vi "CC Pressure Monitor Data buffer.vi"(6 "Clear":bool, 8 "error in (no error)":errorcluster, 9 "Write?":bool, 10 "Data":dbl[](array[numeric]), 11 "Time Stamp":timestamp) -> (0 "error out":errorcluster, 3 "XY Graph":T1(graph))   [LabVIEW 2021]
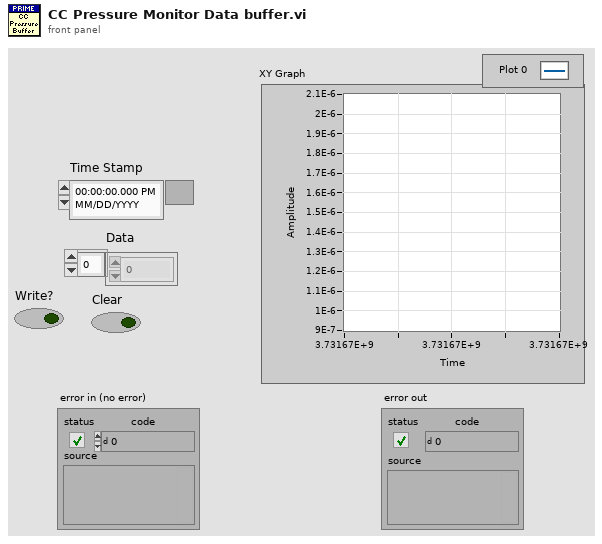
[diagram p1: front panel]
types:
  T1 = cluster{cluster{"Time Stamp":timestamp, "Numeric":dbl}[]}[]
  T2 = cluster{cluster{"Time Stamp":timestamp, "Numeric":dbl}[]}
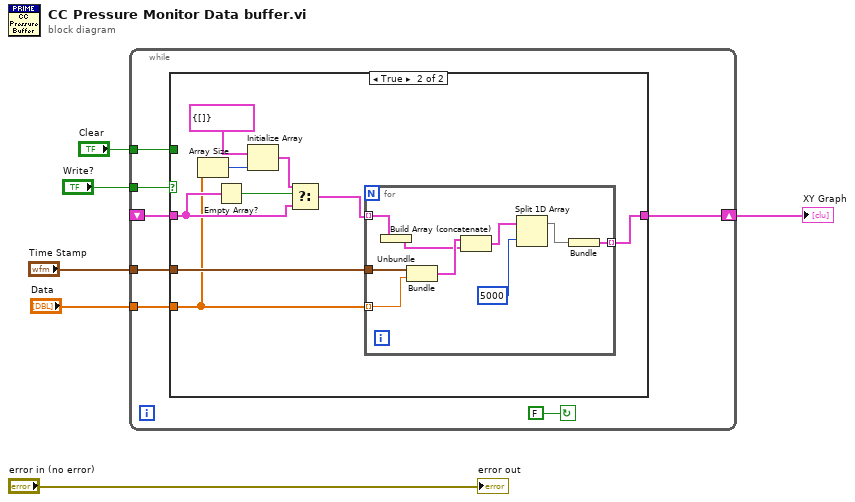
[diagram p0: block diagram]
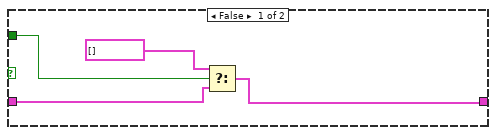
[diagram p2: hidden frame]
diagram:
  n1 = while {
    shift-right: [w9] -> w3
    shift-left: _ -> [w10]
    tunnel: "Data" -> [w12]
    tunnel: "Time Stamp" -> [w11]
    tunnel: "Write?" -> [w8]
    tunnel: "Clear" -> [w7]
    stop <- FALSE continue-if-true
    n2 = case shown="True" w8 {
      tunnel: w12 -> [_ w22]
      tunnel: w11 -> [_ w26]
      tunnel: w10 -> [w14 w24]
      tunnel: [w15 w25] -> w9
      tunnel: w7 -> [w17 _]
      frame False {
        n3 = Select(t=T1 [], s=w17, f=w14) -> (s? t:f=w15:T1)
      }
      frame True {
        n4 = Array Size(array=w22) -> (size(s)=w21:i32)
        n5 = Empty Array?(array=w24) -> (empty?=w18:bool)
        n6 = Initialize Array(T2 {[]}, w21) -> (w19:T1)
        n7 = Select(t=w19, s=w18, f=w24) -> (s? t:f=w23:T1)
        n8 = for {
          tunnel: w23 -> [w35] mode=indexing
          tunnel: w26 -> [w34]
          tunnel: w22 -> [w33] mode=indexing
          tunnel: [w30] -> w25 mode=indexing
          n9 = Unbundle(w35) -> (w31:cluster{"Time Stamp":timestamp, "Numeric":dbl}[])
          n10 = Bundle("Time Stamp"=w34, "Numeric"=w33) -> (w32:cluster{"Time Stamp":timestamp, "Numeric":dbl})  [unwired: 1 in]
          n11 = Build Array (concatenate)(w32, w31) -> (w29:cluster{"Time Stamp":timestamp, "Numeric":dbl}[])
          n12 = Split 1D Array(array=w29, index=5000) -> (first subarray=w27:cluster{"Time Stamp":timestamp, "Numeric":dbl}[])  [unwired: 1 out]
          n13 = Bundle(w27) -> (w30:T2)  [unwired: 1 in]
        }
      }
    }
  }
  "XY Graph" <- w3
  "error out" <- "error in (no error)"
